vi "EMS Device Load Status.vi"(4 "Error String":string, 6 "Status":T1, 8 "error in (no error)":errorcluster, 9 "IED Name":string, 10 "CID Filename":string, 11 "Master Controller in":refnum<class "Master Controller.lvclass">) -> (0 "error out":errorcluster, 3 "Master Controller out":refnum<class "Master Controller.lvclass">)   [LabVIEW 2015, in "Master Controller Core.lvlib" / "Master Controller.lvclass"]
uses:
  Master Controller.lvclass
  SCADA Core/SCADA Abstract Messages/Device Load Status Msg/Device Load Status.ctl
  Communications/SCADA Communcations Actor/SCADA Communications/Controls/EMS Message Cluster.ctl
  Master Controller.lvclass/Master Controller.ctl
  Communications/SCADA Communcations Actor/SCADA Communications Messages/Transmit EMS Message Msg/Transmit EMS Message Msg.lvclass/Transmit EMS Message Msg.ctl
  <vilib>/ActorFramework/Message Enqueuer/Message Enqueuer.lvclass/Message Enqueuer.ctl
  <vilib>/ActorFramework/Message Enqueuer/Enqueue.vi
  <vilib>/ActorFramework/Message Priority Queue/Priority Enqueue.vi
  Communications/SCADA Communcations Actor/SCADA Communications Messages/Transmit EMS Message Msg/Transmit EMS Message Msg.lvclass
  Utilities/Message Strings.llb/Message String Utilities.lvlib
  Communications/SCADA Communcations Actor/SCADA Communications/SCADA Communications.lvclass
  Utilities/Status Messaging.llb/Status Messaging.lvlib
  SCADA Core/SCADA Abstract Messages/Device Load Status Msg/Device Load Status Msg.lvclass
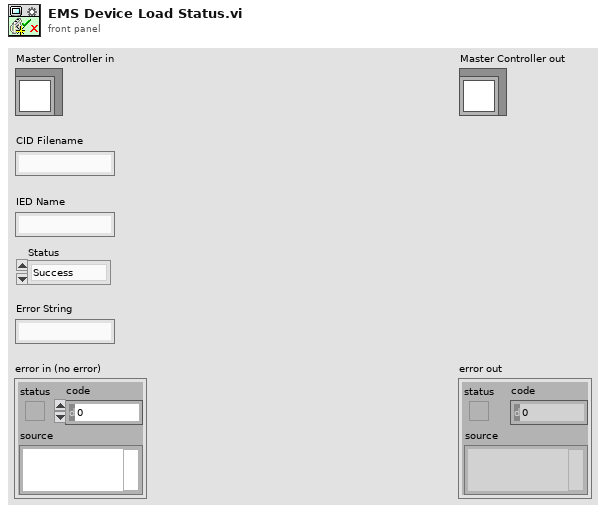
[diagram p1: front panel]
types:
  T1 = typedef "SCADA Core.lvlib/Device Load Status Msg.lvclass/Device Load Status.ctl" = enum16{"Success", "Failure"}
  T2 = typedef "SCADA Communcations Actor.lvlib/SCADA Communications.lvclass/EMS Message Cluster.ctl" = cluster{"Name":string, "Content":string}
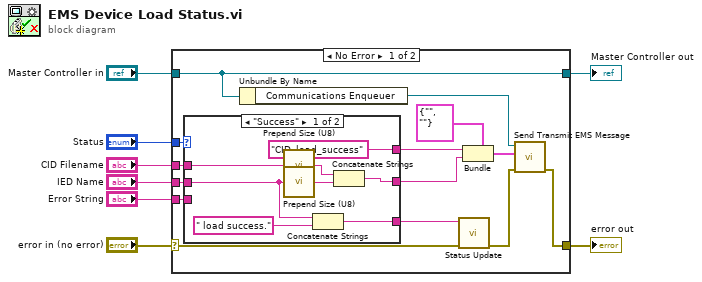
[diagram p0: block diagram]
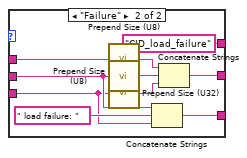
[diagram p2: hidden frame]
diagram:
  n1 = case shown="No Error" "error in (no error)" {
    selector: "error in (no error)" -> [w11 w42]
    tunnel: [w17 w42] -> w7
    tunnel: [w21 w41] -> w5
    tunnel: "Master Controller in" -> [w21 w41]
    tunnel: "IED Name" -> [w14 _]
    tunnel: "Status" -> [w22 _]
    tunnel: "Error String" -> [w15 _]
    tunnel: "CID Filename" -> [w13 _]
    frame No Error {
      n2 = case shown="\"Success\"" w22 {
        tunnel: ["CID_load_success" ("Name") "CID_load_failure" ("Name")] -> w16
        tunnel: w15 -> [_ w32]
        tunnel: w14 -> [w25 w33]
        tunnel: w13 -> [w29 w39]
        tunnel: [w26 w35] -> w12
        tunnel: [w23 w31] -> w9
        frame "Success" {
          n3 = call "Prepend Size (U8).vi"("String in"=w29) -> ("String out"=w28:string)
          n4 = call "Prepend Size (U8).vi"("String in"=w25) -> ("String out"=w27:string)
          n5 = Concatenate Strings(w25, " load success." ("Name")) -> (w23:string)
          n6 = Concatenate Strings(w28, w27) -> (w26:string)
        }
        frame "Failure" {
          n7 = call "Prepend Size (U8).vi"("String in"=w39) -> ("String out"=w37:string)
          n8 = call "Prepend Size (U8).vi"("String in"=w33) -> ("String out"=w38:string)
          n9 = call "Prepend Size (U32).vi"("String in"=w32) -> ("String out"=w36:string)
          n10 = Concatenate Strings(w33, " load failure: " ("Name"), w32) -> (w31:string)
          n11 = Concatenate Strings(w37, w38, w36) -> (w35:string)
        }
      }
      n12 = Unbundle By Name(w21) -> ("Communications Enqueuer"=w19:refnum<class "Message Enqueuer.lvclass">)
      n13 = call "Status Update.vi"("error in (no error)"=w11, "Status Update"=w9) -> ("error out"=w10:errorcluster)  [unwired: 8 in, 1 out]
      n14 = Bundle(cluster=T2 {"Name"="", "Content"=""} ("Message"), "Name"=w16, "Content"=w12) -> (w18:T2)
      n15 = call "Send Transmit EMS Message.vi"("error in (no error)"=w10, "Message"=w18, "Message Enqueuer"=w19) -> ("error out"=w17:errorcluster)  [unwired: 7 in, 1 out]
    }
    frame Error {
    }
  }
  "error out" <- w7
  "Master Controller out" <- w5
